vi "HRR-Command.vi"(8 "error in":errorcluster, 10 "Enable":bool[](array[boolean])) -> (0 "error out":errorcluster, 3 "FPGA VI Reference Out":refnum<k20>)   [LabVIEW 2019]
uses:
  <vilib>/FPGAPlugInAG/myRIO-1900/niLvFpga_Open_myRIO-1900.vi
  <vilib>/rvi/interface/common/dynamic/niFpgaDynamicAddResources.vi
  <vilib>/myRIO/Common/Instrument Driver Framework/Utilities/vis/FPGA Ref Manager.vi
  <vilib>/Utility/error.llb/Error Cluster From Error Code.vi
  <vilib>/myRIO/Common/Instrument Driver Framework/Utilities/vis/Ref Counter.vi
  <vilib>/rvi/interface/common/niFpgaWaitOnOcc.vi
  <vilib>/rvi/interface/nirviOpenFPGA/nirviOpenFPGA.xnode
  FPGA Bitfiles/MyRIOFPGATest_FPGATarget_FPGAMainDefault_pJ5Q7Xj1Ujo.lvbitx
  FPGA Main Default.vi
  <vilib>/rvi/interface/nirviMethod/nirviMethod.xnode
  <vilib>/FPGAPlugInAG/Dynamic/niLvFpga_ConfigureFifo_Dynamic.vi
  <vilib>/rvi/errors/niLvFpgaMergeErrorWithErrorCode.vi
  <vilib>/myRIO/Instrument Drivers/Utilities/Utilities.lvlib
panel:
  out "Actual Depth":u32
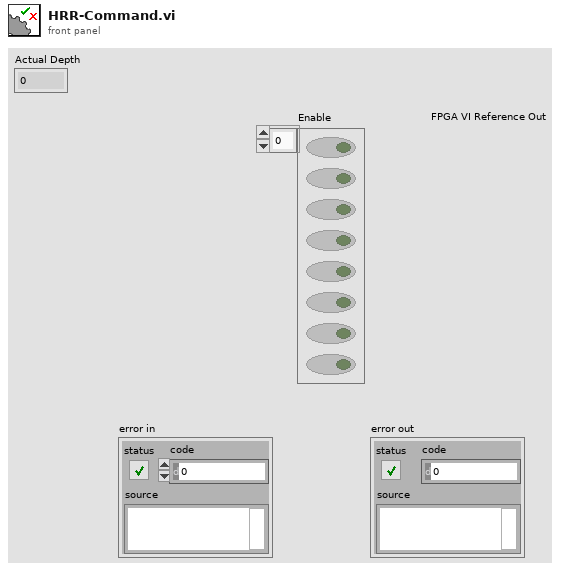
[diagram p1: front panel]
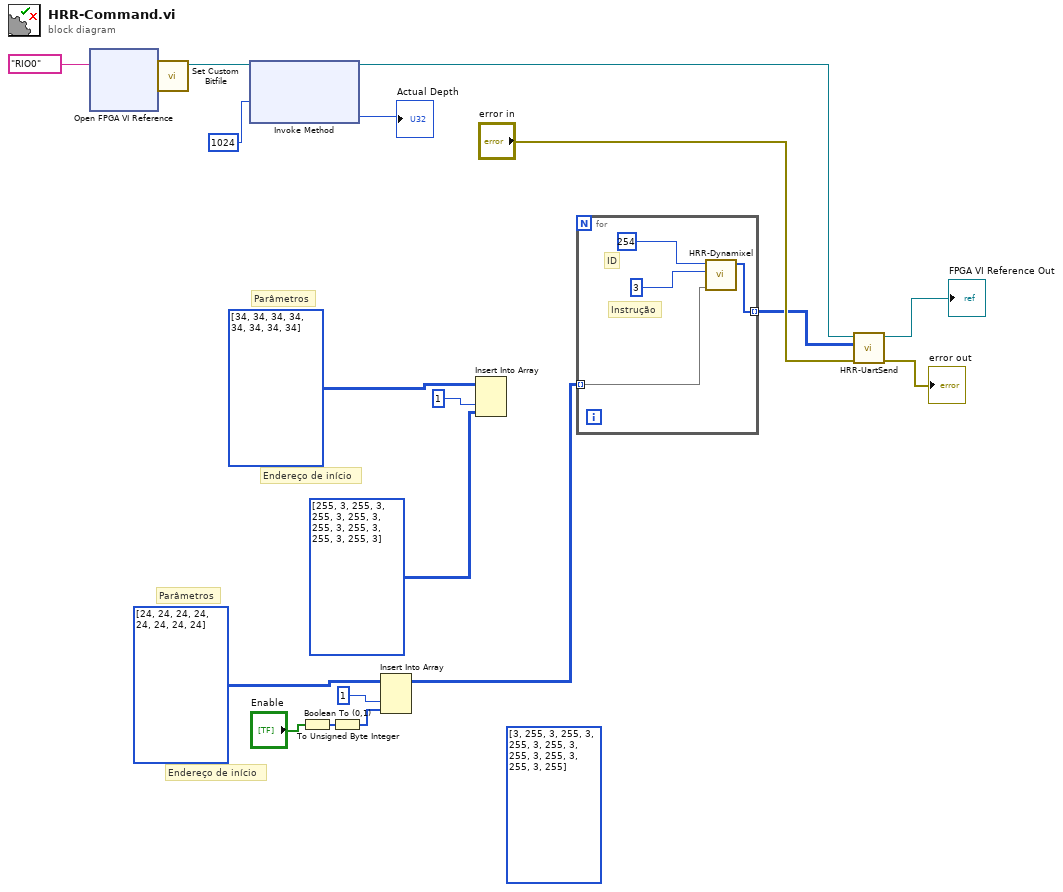
[diagram p0: block diagram]
diagram:
  (unwired) u8[][] [[3, 255], [3, 255], [3, 255], [3, 255], [3, 255], [3, 255], [3, 255], [3, 255]] ("array")
  # "Parâmetros"
  # "Endereço de início"
  # "Parâmetros"
  # "Endereço de início"
  n1 = xnode "Open FPGA VI Reference"("resource name"=tag "RIO0") -> ("FPGA VI Reference Out"=w7:refnum<k20>, "error out"=w8:errorcluster)  [unwired: 1 in]
  n2 = call <vilib>:"Set Custom Bitfile.vi"("error in (no error)"=w8, "Custom FPGA Reference In"=w7) -> ("Custom FPGA Reference Out"=w6:refnum<k20>)  [unwired: 8 in, 1 out]
  n3 = xnode "Invoke Method"("FPGA VI Reference In"=w6, "Requested Depth"=u32 1024) -> ("FPGA VI Reference Out"=w5:refnum<k20>, "Actual Depth"=→"Actual Depth":u32)  [unwired: 1 in, 1 out]
  n4 = Boolean To (0,1)(Boolean="Enable") -> (0, 1=w13:i16[])
  n5 = To Unsigned Byte Integer(number=w13) -> (unsigned 8bit integer=w12:u8[])
  n6 = Insert Into Array(array=u8[][] [[24], [24], [24], [24], [24], [24], [24], [24]], index (col)=1 ("disabled index (col)"), new element=w12) -> (w1:u8[][])  [unwired: 1 in]
  n7 = Insert Into Array(array=u8[][] [[34], [34], [34], [34], [34], [34], [34], [34]], index (col)=1 ("disabled index (col)"), new element=u8[][] [[255, 3], [255, 3], [255, 3], [255, 3], [255, 3], [255, 3], [255, 3], [255, 3]] ("array")) -> ()  [unwired: 1 in, 1 out]
  n8 = for {
    tunnel: [w22] -> w15 mode=indexing
    tunnel: w1 -> [w21] mode=indexing
    # "Instrução"
    # "ID"
    n9 = call "HRR-Dynamixel.vi"("ID"=u8 254, "Instruction"=u8 3, "Array in"=w21) -> ("Array out"=w22:u8[])  [unwired: 7 in]
  }
  n10 = call "HRR-UartSend.vi"("error in (no error)"="error in", "Array"=w15, "Refnum in"=w5) -> ("error out"=→"error out":errorcluster, "Refnum out"=→"FPGA VI Reference Out":refnum<k20>)  [unwired: 7 in]
